vi "Init AI DAQ v2.vi"(8 "error in":errorcluster, 10 "DAQChan[]":T1[](array[typedef]), 11 "TaskName":string="AI Task") -> (0 "error out":errorcluster, 3 "AI TaskRef":refnum<k21>)   [LabVIEW 2017]
doc: "Developed by Kevin Thompson\nThompson Engineering, LLC\nkevin@thompsonengineering.net"
uses:
  Analog DAQChan--cluster.ctl
  AI InstrType--enum.ctl
  <vilib>/DAQmx/create/channels.llb/DAQmx Create Channel (AI-Voltage-Basic).vi
  <vilib>/DAQmx/create/channels.llb/DAQmx Create Channel (AI-Current-Basic).vi
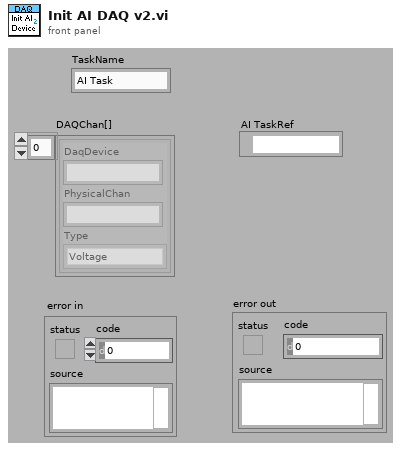
[diagram p1: front panel]
types:
  T1 = typedef "Analog DAQChan--cluster.ctl" = cluster{"DaqDevice":string, "PhysicalChan":string, "Type":T2}
  T2 = typedef "AI InstrType--enum.ctl" = enum16{"Voltage", "Current"}
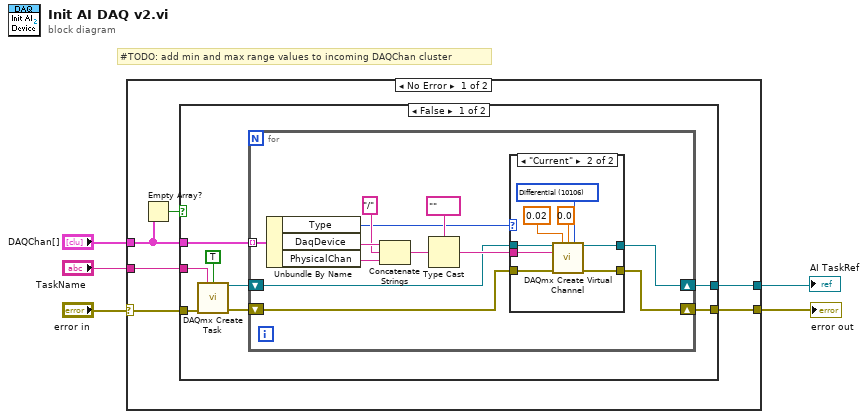
[diagram p0: block diagram]
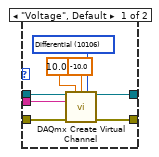
[diagram p2: hidden frame]
diagram:
  # "#TODO: add min and max range values to incoming DAQChan cluster"
  n1 = case shown="No Error" "error in" {
    selector: "error in" -> [w9 w49]
    tunnel: "DAQChan[]" -> [w6 _]
    tunnel: [w11 _] -> w4
    tunnel: [w10 w49] -> w3
    tunnel: "TaskName" -> [w8 _]
    frame No Error {
      n2 = Empty Array?(array=w6) -> (empty?=w7:bool)
      n3 = case shown="False" w7 {
        tunnel: w6 -> [w19 _]
        tunnel: [w15 _] -> w11
        tunnel: [w14 w48] -> w10
        tunnel: w9 -> [w13 w48]
        tunnel: w8 -> [w12 _]
        frame False {
          n4 = call <vilib>:"DAQmx Create Task.vi"("new task name"=w12, "auto cleanup"=TRUE, "error in"=w13) -> ("task out"=w17:refnum<k21>, "error out"=w16:errorcluster)  [unwired: 11 in]
          n5 = for {
            tunnel: w19 -> [w31] mode=indexing
            shift-right: [w23] -> w15
            shift-left: w17 -> [w24]
            shift-right: [w20] -> w14
            shift-left: w16 -> [w21]
            n6 = Unbundle By Name(w31) -> ("Type"=w22:T2, "DaqDevice"=w30:string, "PhysicalChan"=w28:string)
            n7 = Concatenate Strings(w30, "/", w28) -> (w26:string)
            n8 = Type Cast(type=tag "" ("PhysChan"), x=w26) -> (*(type *) &x=w25:tag)
            n9 = case shown="\"Current\"" w22 {
              tunnel: w24 -> [w39 w47]
              tunnel: w25 -> [w38 w46]
              tunnel: w21 -> [w34 w42]
              tunnel: [w33 w41] -> w20
              tunnel: [w32 w40] -> w23
              frame "Voltage", Default {
                w37 = 10106 items=["default"=-1, "RSE"=10083, "NRSE"=10078, "Differential"=10106, "Pseudodifferential"=12529] ("termConfig")
                n10 = call-poly <vilib>:"DAQmx Create Virtual Channel.vi"("task in"=w39, "maximum value"=10.0 ("maxValue"), "minimum value"=-10.0 ("minValue"), "input terminal configuration"=w37, "physical channels"=w38, "error in"=w34) -> ("task out"=w32:refnum<k21>, "error out"=w33:errorcluster)  [unwired: 8 in]
              }
              frame "Current" {
                w45 = 10106 items=["default"=-1, "RSE"=10083, "NRSE"=10078, "Differential"=10106, "Pseudodifferential"=12529] ("termConfig")
                n11 = call-poly <vilib>:"DAQmx Create Virtual Channel.vi"("task in"=w47, "maximum value"=0.02 ("maxValue"), "minimum value"=0.0 ("minValue"), "input terminal configuration"=w45, "physical channels"=w46, "error in"=w42) -> ("task out"=w40:refnum<k21>, "error out"=w41:errorcluster)  [unwired: 8 in]
              }
            }
          }
        }
        frame True {
        }
      }
    }
    frame Error {
    }
  }
  "AI TaskRef" <- w4
  "error out" <- w3
